vi "Get Step Config.vi"(0 "VI In":refnum<vi>, 11 "error in":errorcluster) -> (4 "VI out":refnum<vi>, 6 "Wash Array":T1[](array[typedef]), 15 "error out":errorcluster)   [LabVIEW 2016]
uses:
  Controls/Wash Step Config.ctl
  <vilib>/Utility/config.llb/Read Key (U32).vi
  <vilib>/Utility/config.llb/Read Key (Double).vi
  <vilib>/Utility/config.llb/NI_LVConfig.lvlib
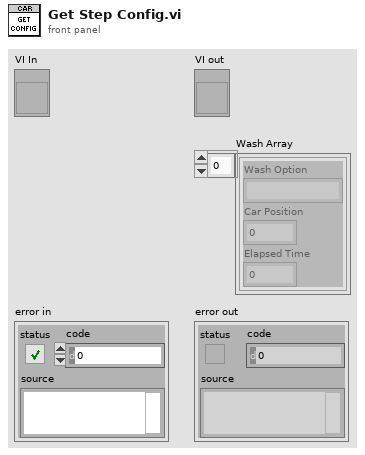
[diagram p1: front panel]
types:
  T1 = typedef "Wash Step Config.ctl" = cluster{"Wash Option":string, "Car Position":u8, "Elapsed Time":dbl}
  T2 = typedef "NI_LVConfig.lvlib/Config Data RefNum.ctl" = refnum<k1>
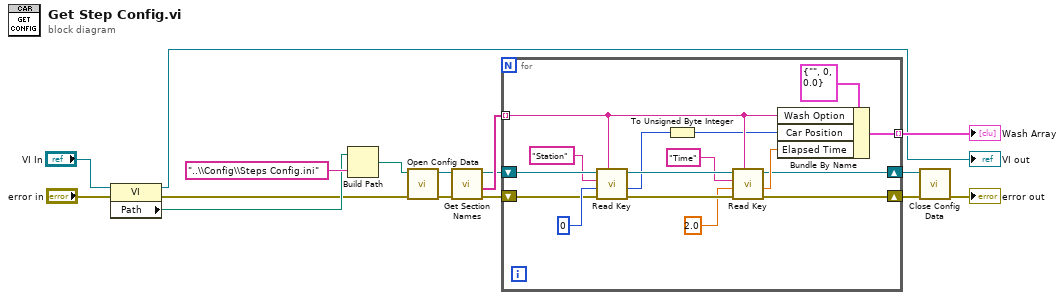
[diagram p0: block diagram]
diagram:
  n1 = property class="VI"(reference="VI In", error in="error in") -> (reference out=→"VI out":refnum<vi>, error out=w1:errorcluster, "Path"=w2:path)
  n2 = Build Path(base path=w2, name or relative path="..\\Config\\Steps Config.ini") -> (appended path=w4:path)
  n3 = call <vilib>:"Open Config Data.vi"("error in (no error)"=w1, "configuration file path"=w4) -> ("error out"=w6:errorcluster, "refnum"=w5:T2)  [unwired: 7 in, 1 out]
  n4 = call <vilib>:"Get Section Names.vi"("error in (no error)"=w6, "refnum"=w5) -> ("error out"=w9:errorcluster, "section names"=w8:string[], "refnum out"=w7:T2)  [unwired: 7 in]
  n5 = for {
    tunnel: w8 -> [w25] mode=indexing
    tunnel: [w21] -> w16 mode=indexing
    shift-right: [w20] -> w10
    shift-left: w9 -> [w29]
    shift-right: [w19] -> w11
    shift-left: w7 -> [w31]
    n6 = call-poly <vilib>:"Read Key.vi"("section"=w25, "error in (no error)"=w29, "default value"=u32 0, "key"="Station", "refnum"=w31) -> ("error out"=w27:errorcluster, "value"=w24:u32, "refnum out"=w28:T2)  [unwired: 3 in, 1 out]
    n7 = To Unsigned Byte Integer(number=w24) -> (unsigned 8bit integer=w22:u8)
    n8 = call-poly <vilib>:"Read Key.vi"("section"=w25, "error in (no error)"=w27, "default value"=2.0, "key"="Time", "refnum"=w28) -> ("error out"=w20:errorcluster, "value"=w23:dbl, "refnum out"=w19:T2)  [unwired: 3 in, 1 out]
    n9 = Bundle By Name(cluster=T1 {"Wash Option"="", "Car Position"=0, "Elapsed Time"=0.0}, "Wash Option"=w25, "Car Position"=w22, "Elapsed Time"=w23) -> (w21:T1)
  }
  "Wash Array" <- w16
  n10 = call <vilib>:"Close Config Data.vi"("error in (no error)"=w10, "refnum"=w11) -> ("error out"=→"error out":errorcluster)  [unwired: 8 in, 1 out]
